vi "Configure Digitize Voltage.vi"(0 "VISA resource name":refnum<visa-resource-name>, 1 "AC Filter Type":u16(ring) items=["Slow", "Fast"], 5 "Manual Range":dbl=10.0, 7 "Aperture Seconds":dbl=0.01616 min=8.333e-06 max=0.25 step=1e-06, 9 "Coupling":u16(ring)=1 items=["AC", "DC"], 11 "error in (no error)":errorcluster, 12 "Filter Frequency":dbl=1000.0) -> (4 "VISA resource name out":refnum<visa-resource-name>, 15 "error out":errorcluster)   [LabVIEW 2018, in "Keithley DMM7512.lvlib"]
doc: "This VI configures the Digitize Voltage and the related parameters."
uses:
  <instrlib>/Keithley DMM7512/Keithley DMM7512.lvlib
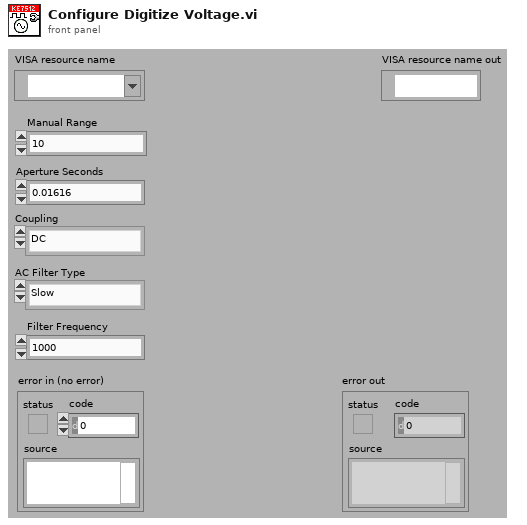
[diagram p1: front panel]
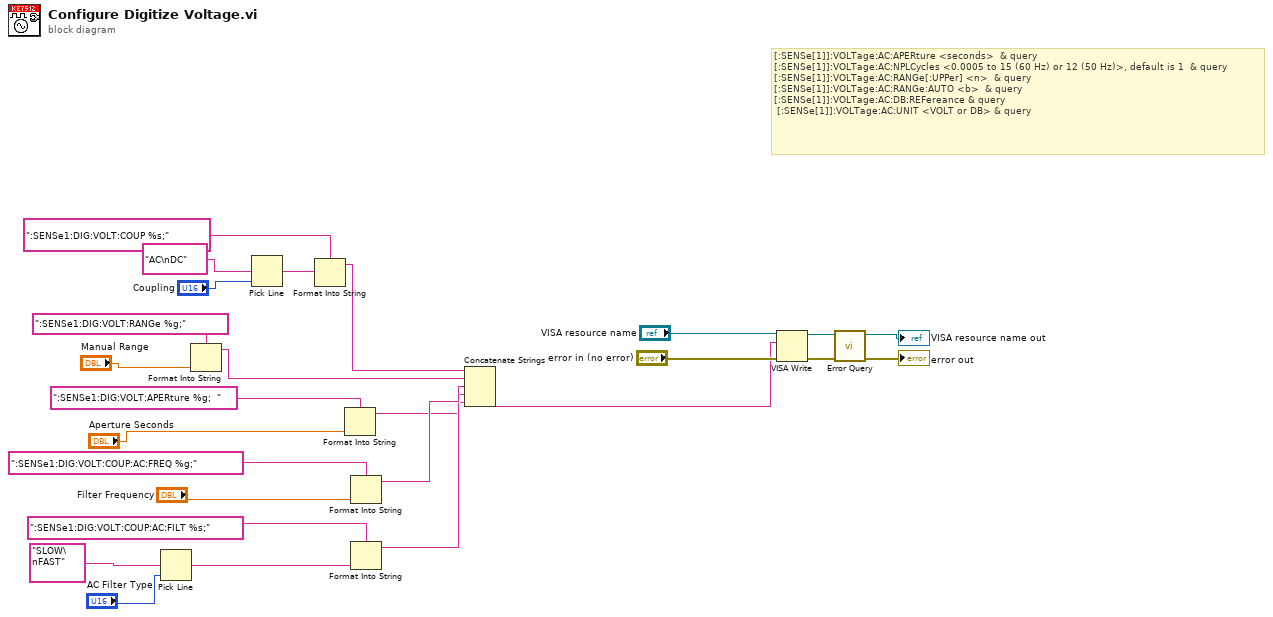
[diagram p0: block diagram]
diagram:
  # "[:SENSe[1]]:VOLTage:AC:APERture <seconds>  & query\n[:SENSe[1]]:VOLTage:AC:NPLCycles <0.0005 to 15 (60 Hz) or 12 (50 Hz)>, default is 1  & query\n[:SENSe[1]]:VOLTage:AC:RANGe[:UPPer] <n>  & query\n[:SENSe[1]]:VOLTage:AC:RANGe:AUTO <b>  & query\n[:SENSe[1]]:VOLTage:AC:DB:REFereance & query\n [:SENSe[1]]:VOLTage:AC:UNIT <VOLT or DB> & query"
  n1 = Pick Line(multi-line string="SLOW\nFAST", line index="AC Filter Type") -> (output string=w16:string)  [unwired: 1 in]
  n2 = Format Into String(format string=":SENSe1:DIG:VOLT:RANGe %g;", "Manual Range") -> (resulting string=w3:string)  [unwired: 2 in, 1 out]
  n3 = Pick Line(multi-line string="AC\nDC", line index="Coupling") -> (output string=w7:string)  [unwired: 1 in]
  n4 = Format Into String(format string=":SENSe1:DIG:VOLT:COUP %s;", w7) -> (resulting string=w21:string)  [unwired: 2 in, 1 out]
  n5 = Format Into String(format string=":SENSe1:DIG:VOLT:APERture %g;  ", "Aperture Seconds") -> (resulting string=w1:string)  [unwired: 2 in, 1 out]
  n6 = Format Into String(format string=":SENSe1:DIG:VOLT:COUP:AC:FREQ %g;", "Filter Frequency") -> (resulting string=w14:string)  [unwired: 2 in, 1 out]
  n7 = Format Into String(format string=":SENSe1:DIG:VOLT:COUP:AC:FILT %s;", w16) -> (resulting string=w13:string)  [unwired: 2 in, 1 out]
  n8 = Concatenate Strings(w21, w3, w14, w13, w1) -> (w20:string)
  n9 = VISA Write(VISA resource name="VISA resource name", write buffer=w20, error in (no error)="error in (no error)") -> (VISA resource name out=w12:refnum<visa-resource-name>, error out=w11:errorcluster)  [unwired: 1 out]
  n10 = call <instrlib>:"Error Query.vi"("error in (no error)"=w11, "VISA resource name"=w12) -> ("error out"=→"error out":errorcluster, "VISA resource name out"=→"VISA resource name out":refnum<visa-resource-name>)  [unwired: 6 in, 2 out]
